vi "Send Stop Nested Actors.vi"(8 "error in (no error)":errorcluster, 9 "Message Priority (Normal)":T1=enum."Normal", 11 "Message Enqueuer":refnum<class "Message Enqueuer.lvclass">) -> (0 "error out":errorcluster, 3 "Message Enqueuer out":refnum<class "Message Enqueuer.lvclass">)   [LabVIEW 2020, in "Actor with Nesteds.lvlib" / "Stop Nested Actors Msg.lvclass"]
doc: "<p>(<strong>Filename</strong>: <span class=\"dnl\">Actor Framework.lvlib:Report Error Msg.lvclass:Send Error Report.vi</span>)</p>\n\n<p>Use this VI to send an error to an actor. The error will be handled by the Handle Error VI of the actor. If the error is not handled there, it will cause the actor to stop running.</p>"
uses:
  Stop Nested Actors Msg.lvclass
  ActorFramework/Message Enqueuer/Message Enqueuer.lvclass
  ActorFramework/Message Enqueuer/Message Priority.ctl
  C:/justACS/Actor Framework/Core/ActorFramework/Message/Message.lvclass
  ActorFramework/Message Enqueuer/Message Enqueuer.lvclass/Message Enqueuer.ctl
  ActorFramework/Message Priority Queue/Priority Enqueue.vi
  Stop Nested Actors Msg.lvclass/Stop Nested Actors Msg.ctl
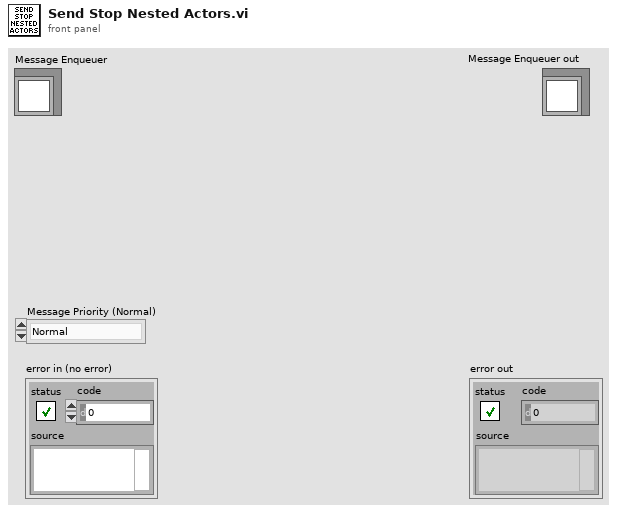
[diagram p1: front panel]
types:
  T1 = typedef "Actor Framework.lvlib/Message Enqueuer.lvclass/Message Priority.ctl" = enum16{"Low", "Normal", "High"}
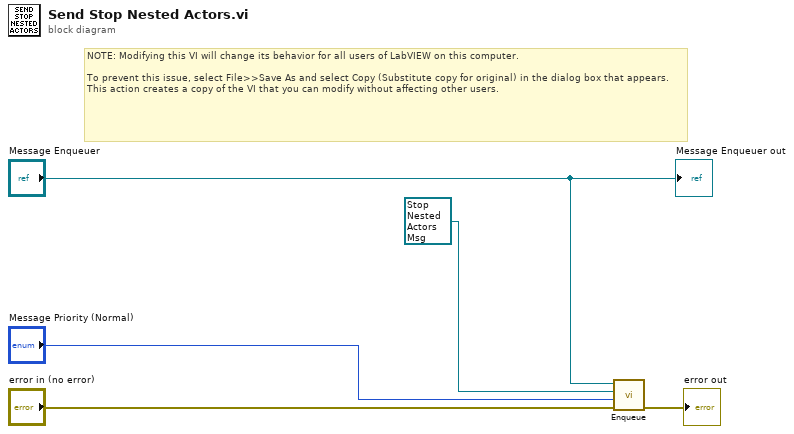
[diagram p0: block diagram]
diagram:
  # "NOTE: Modifying this VI will change its behavior for all users of LabVIEW on this computer.\n\nTo prevent this issue, select File>>Save As and select Copy (Substitute copy for original) in the dialog box that appears. This action creates a copy of the VI that you can modify without affecting other users."
  n1 = call "Enqueue.vi"("error in (no error)"="error in (no error)", "Message Priority (Normal)"="Message Priority (Normal)", "Message"=refnum<class "Stop Nested Actors Msg.lvclass"> refnum ("Report Error Msg in"), "Message Enqueuer in"="Message Enqueuer") -> ("error out"=→"error out":errorcluster)  [unwired: 6 in, 1 out]
  "Message Enqueuer out" <- "Message Enqueuer"
